vi "Set FIFO Overflow Error.vi"(0 "fifo name":string, 5 "overflow":bool, 11 "error in (no error)":errorcluster) -> (15 "error out":errorcluster)   [LabVIEW 2023, in "GettingStarted_Common_148X_Host.lvlib"]
uses:
  GettingStarted_Common_148X_Host.lvlib
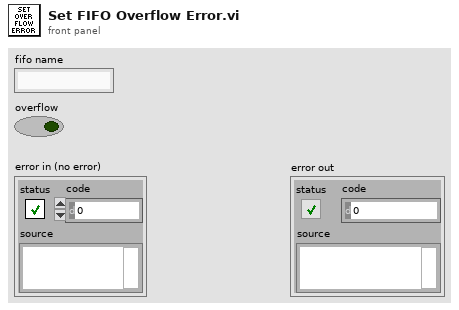
[diagram p1: front panel]
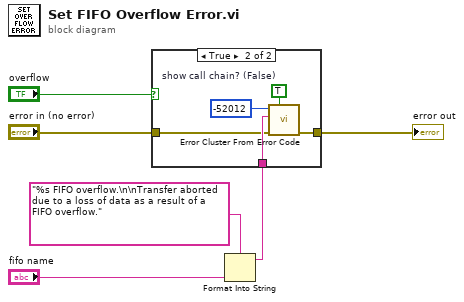
[diagram p0: block diagram]
diagram:
  n1 = Format Into String(format string="%s FIFO overflow.\n\nTransfer aborted due to a loss of data as a result of a FIFO overflow.", "fifo name") -> (resulting string=w6:string)  [unwired: 2 in, 1 out]
  n2 = case shown="True" "overflow" {
    tunnel: [w7 w12] -> w5
    tunnel: w6 -> [_ w9]
    tunnel: "error in (no error)" -> [w7 w8]
    frame False {
    }
    frame True {
      w11 = TRUE  # show call chain? (False)
      n3 = call <vilib>:"Error Cluster From Error Code.vi"("show call chain? (False)"=w11, "error in (no error)"=w8, "error message (\"\")"=w9, "error code (0)"=-52012) -> ("error out"=w12:errorcluster)  [unwired: 5 in]
    }
  }
  "error out" <- w5
